vi "Launch Nested.vi"(8 "error in (no error)":errorcluster, 9 "Actor":refnum<class "Actor.lvclass">, 10 "Name":string, 11 "MVVM Abstruct Model in":refnum<class "MVVM Abstruct Model.lvclass">) -> (0 "error out":errorcluster, 3 "MVVM Abstruct Model out":refnum<class "MVVM Abstruct Model.lvclass">)   [LabVIEW 2020, in "MVVM Abstruct Model.lvlib" / "MVVM Abstruct Model.lvclass"]
uses:
  MVVM Abstruct Model.lvclass
  C:/Program Files (x86)/National Instruments/LabVIEW 2020/vi.lib/ActorFramework/Actor/Actor.lvclass
  <vilib>/ActorFramework/Actor/Actor.lvclass
  <vilib>/ActorFramework/Message/Message.lvclass
  MVVM Abstruct Model.lvclass/MVVM Abstruct Model.ctl
  <vilib>/ActorFramework/Actor/Actor.lvclass/Actor.ctl
  <vilib>/ActorFramework/Message Enqueuer/Message Enqueuer.lvclass/Message Enqueuer.ctl
  Enqueues Data/Enqueues Data.lvclass
  Enqueues Data/Enqueues Data.lvclass/Enqueues Data.ctl
  MVVM Abstruct Controller/MVVM Abstruct Controller Messages/Add & Register Models Msg/Add & Register Models Msg.lvclass/Add & Register Models Msg.ctl
  Enqueues Data/Accessors/Write ActorMap.vi
  MVVM Abstruct Controller/MVVM Abstruct Controller Messages/Add & Register Models Msg/Add & Register Models Msg.lvclass
  C:/Program Files (x86)/National Instruments/LabVIEW 2020/vi.lib/ActorFramework/Message/Message.lvclass
  <vilib>/ActorFramework/Message Priority Queue/Priority Enqueue.vi
  C:/Users/yu/Desktop/Pro1/06 Source/Code/Common/ActorMap/ActorMap.lvclass
  <vilib>/ActorFramework/Message Enqueuer/Message Enqueuer.lvclass
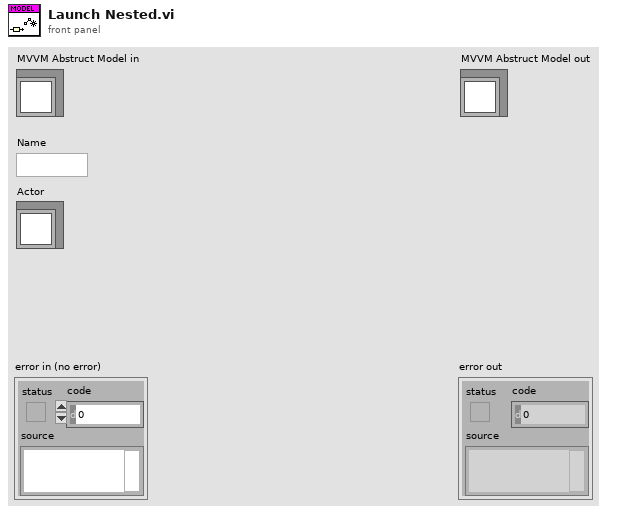
[diagram p1: front panel]
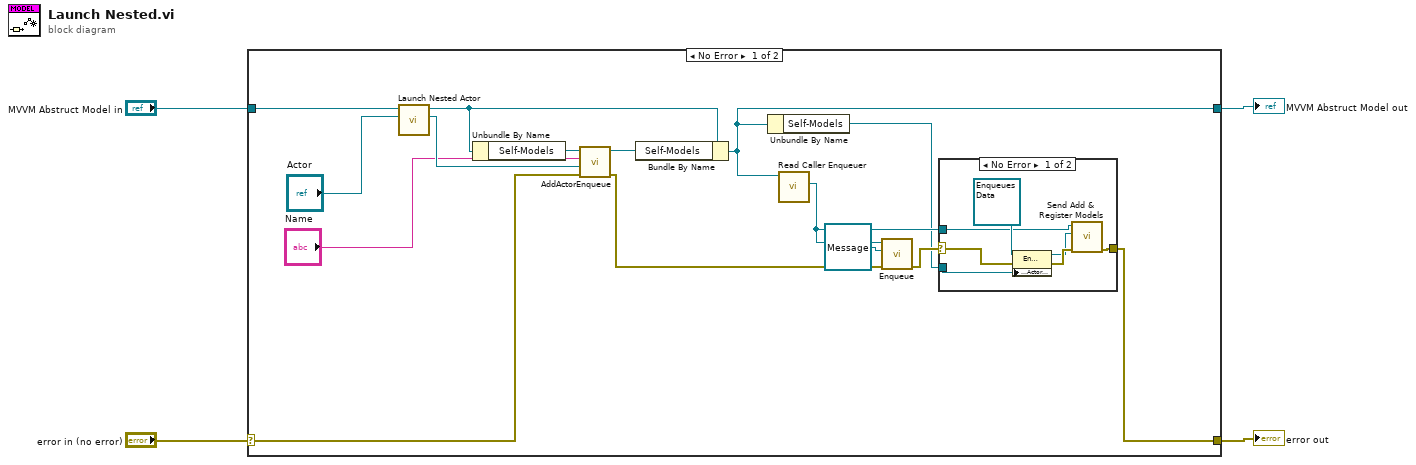
[diagram p0: block diagram]
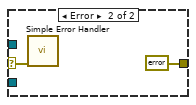
[diagram p2: hidden frame]
diagram:
  n1 = case shown="No Error" "error in (no error)" {
    selector: "error in (no error)" -> [w12 w30]
    tunnel: [w5 w30] -> w3
    tunnel: [w6 w29] -> w1
    tunnel: "MVVM Abstruct Model in" -> [w19 w29]
    frame No Error {
      n2 = call <vilib>:"Launch Nested Actor.vi"("Nested Actor"="Actor", "Caller Actor in"=w19) -> ("Nested Actor's Enqueuer"=w14:refnum<class "Message Enqueuer.lvclass">, "Caller Actor out"=w17:refnum<class "MVVM Abstruct Model.lvclass">)  [unwired: 7 in, 1 out]
      n3 = Unbundle By Name(w17) -> ("Self-Models"=w16:refnum<class "ActorMap.lvclass">)
      n4 = call "AddActorEnqueue.vi"("error in (no error)"=w12, "Actor's Enqueuer"=w14, "name"="Name", "ActorMap in"=w16) -> ("error out"=w7:errorcluster, "ActorMap out"=w15:refnum<class "ActorMap.lvclass">)  [unwired: 6 in]
      n5 = Bundle By Name(cluster=w17, "Self-Models"=w15) -> (w6:refnum<class "MVVM Abstruct Model.lvclass">)
      n6 = Unbundle By Name(w6) -> ("Self-Models"=w8:refnum<class "ActorMap.lvclass">)
      n7 = call <vilib>:"Read Caller Enqueuer.vi"("Actor"=w6) -> ("Caller Enqueuer"=w9:refnum<class "Message Enqueuer.lvclass">)  [unwired: 10 in]
      n8 = call <vilib>:"Enqueue.vi"("error in (no error)"=w7, "Message"=refnum<class "Message.lvclass"> refnum, "Message Enqueuer in"=w9) -> ("error out"=w10:errorcluster)  [unwired: 7 in, 1 out]
      n9 = case shown="No Error" w10 {
        selector: w10 -> [w24 w28]
        tunnel: [w21 errorcluster {"status"=FALSE, "code"=0, "source"=""} ("error out")] -> w5
        tunnel: w9 -> [w23 _]
        tunnel: w8 -> [w25 _]
        frame No Error {
          n10 = property class="Enqueues Data.lvclass"(reference=refnum<class "Enqueues Data.lvclass"> refnum ("View"), error in=w24, "Accessors:ActorMap"=w25) -> (reference out=w20:refnum<class "Enqueues Data.lvclass">, error out=w22:errorcluster)
          n11 = call "Send Add & Register Models.vi"("error in (no error)"=w22, "Models"=w20, "Message Enqueuer"=w23) -> ("error out"=w21:errorcluster)  [unwired: 7 in, 1 out]
        }
        frame Error {
          n12 = call <vilib>:"Simple Error Handler.vi"("error in (no error)"=w28) -> ()  [unwired: 4 in, 5 out]
        }
      }
    }
    frame Error {
    }
  }
  "error out" <- w3
  "MVVM Abstruct Model out" <- w1
